vi "KE6221 -- Arm Waveform Func.vi"(0 "Resource In":refnum<visa-resource-name>, 1 "Check For SCPI Errors? (T)":bool=TRUE, 7 "Wave Type":T1, 11 "error in (no error)":errorcluster) -> (4 "Resource Out (dupl)":refnum<visa-resource-name>, 15 "error out":errorcluster)   [LabVIEW 2019, in "Keithley 622x.lvlib"]
doc: "Arms the selected waveform type for the 6221 (sine, square, ramp, or arbitrary waveform). It also optionally starts playback of the armed waveform."
uses:
  Keithley 622x.lvlib
  Configure/6221 Wave/Low Level/Typedefs/KE6221 -- Wave Type.ctl
panel:
  in  "Init Sweep? (T)":bool=TRUE
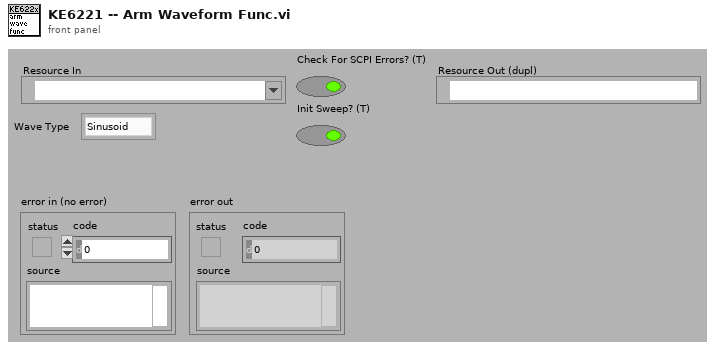
[diagram p1: front panel]
types:
  T1 = typedef "Keithley 622x.lvlib/KE6221 -- Wave Type.ctl" = enum16{"Sinusoid", "Square", "Ramp", "Arbitrary 0", "Arbitrary 1", "Arbitrary 2", "Arbitrary 3", "Arbitrary 4"}
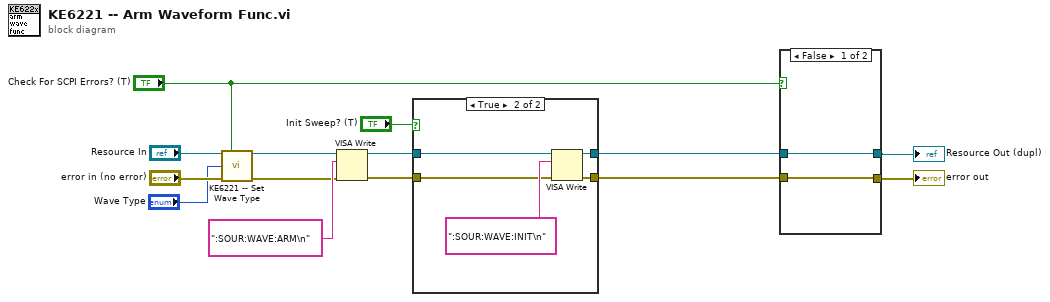
[diagram p0: block diagram]
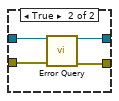
[diagram p3: hidden frame]
diagram:
  n1 = call "KE6221 -- Set Wave Type.vi"("Resource In"="Resource In", "Check For SCPI Errors? (T)"="Check For SCPI Errors? (T)", "Wave Type"="Wave Type", "error in (no error)"="error in (no error)") -> ("Resource Out (dupl)"=w1:refnum<visa-resource-name>, "error out"=w4:errorcluster)  [unwired: 10 in]
  n2 = VISA Write(VISA resource name=w1, write buffer=":SOUR:WAVE:ARM\n" ("format string"), error in (no error)=w4) -> (VISA resource name out=w11:refnum<visa-resource-name>, error out=w8:errorcluster)  [unwired: 1 out]
  n3 = case shown="True" "Init Sweep? (T)" {
    tunnel: w11 -> [w16 w21]
    tunnel: [w16 w19] -> w10
    tunnel: [w15 w18] -> w9
    tunnel: w8 -> [w15 w17]
    frame False {
    }
    frame True {
      n4 = VISA Write(VISA resource name=w21, write buffer=":SOUR:WAVE:INIT\n", error in (no error)=w17) -> (VISA resource name out=w19:refnum<visa-resource-name>, error out=w18:errorcluster)  [unwired: 1 out]
    }
  }
  n5 = case shown="False" "Check For SCPI Errors? (T)" {
    tunnel: w10 -> [w23 w27]
    tunnel: w9 -> [w22 w26]
    tunnel: [w22 w25] -> w12
    tunnel: [w23 w24] -> w13
    frame False {
    }
    frame True {
      n6 = call "Error Query.vi"("VISA Resource In"=w27, "error in (no error)"=w26) -> ("VISA Resource Out (dupl)"=w24:refnum<visa-resource-name>, "error out"=w25:errorcluster)  [unwired: 10 in, 2 out]
    }
  }
  "Resource Out (dupl)" <- w13
  "error out" <- w12
